vi "Accumet 50 Serial Port Init.vi"(1 "flow control etc.":T1={"input XON/XOFF"=FALSE, "input HW Handshake"=FALSE, "input alt HW HShk"=FALSE, "output XON/XOFF"=FALSE, "output HW Handshake"=FALSE, "output alt HW HShk"=FALSE, "XOFF byte "=19, "XON byte"=17, "parity error byte"=0} {"parity error byte" format="%.0x"; "XON byte" format="%.0x"; "XOFF byte" format="%.0x"}, 2 "parity":u16(ring) items=["no parity", "odd parity", "even parity", "mark parity", "space parity"], 3 "buffer size":u16=10000, 4 "stop bits":u16(ring) items=["1 bit", "1.5 bits", "2 bits"], 5 "data bits":u16=8 min=5 max=8 step=1, 6 "baud rate":u16=9600, 7 "port number":i32=1) -> (0 "error code":i32)   [LabVIEW 2010]
doc: "Initializes the selected serial port to the specified settings."
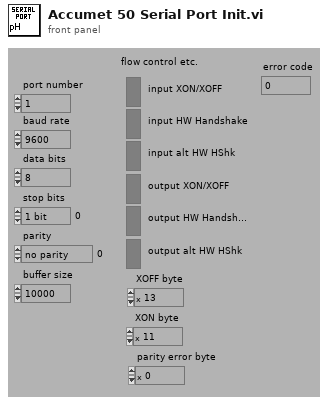
[diagram p1: front panel]
types:
  T1 = cluster{"input XON/XOFF":bool, "input HW Handshake":bool, "input alt HW HShk":bool, "output XON/XOFF":bool, "output HW Handshake":bool, "output alt HW HShk":bool, "XOFF byte ":u8, "XON byte":u8, "parity error byte":u16}
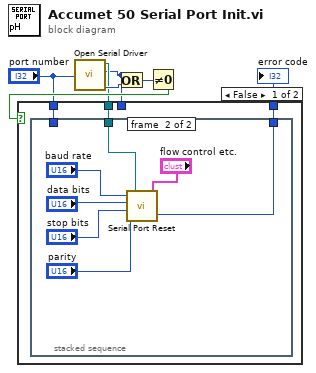
[diagram p0: block diagram]
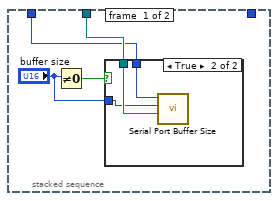
[diagram p2: hidden frame]
diagram:
  n1 = call <vilib>:"Open Serial Driver.vi"("port number"="port number") -> ("input refnum"=w4:refnum<visa-resource-name>, "input error"=w2:i32, "output error"=w6:i32)  [unwired: 1 out]
  n2 = Or(x=w2, y=w6) -> (x .or. y?=w7:i32)
  n3 = Not Equal To 0?(x=w7) -> (x != 0?=w5:bool)
  n4 = case shown="False" w5 {
    tunnel: w4 -> [w10 _]
    tunnel: [w9 w25] -> w3
    tunnel: w2 -> [_ w25]
    tunnel: "port number" -> [w8 _]
    frame False {
      n5 = stacked-sequence {
        tunnel: w10 -> [w12 w24]
        tunnel: [_ w20] -> w9
        tunnel: w8 -> [w11 _]
        frame #0 {
          n6 = Not Equal To 0?(x="buffer size") -> (x != 0?=w14:bool)
          n7 = case shown="True" w14 {
            tunnel: "buffer size" -> [_ w16]
            tunnel: w12 -> [_ w17]
            tunnel: w11 -> [_ w15]
            frame False {
            }
            frame True {
              n8 = call <vilib>:"Serial Port Buffer Size.vi"("in ref"=w17, "buffer size"=w16, "port number (unused)"=w15) -> ()  [unwired: 1 in, 1 out]
            }
          }
        }
        frame #1 {
          n9 = call <vilib>:"Serial Port Reset.vi"("flow control etc."="flow control etc.", "input refnum"=w24, "parity"="parity", "stop bits"="stop bits", "data bits"="data bits", "baud rate"="baud rate") -> ("error"=w20:i32)  [unwired: 1 in]
        }
      }
    }
    frame True {
    }
  }
  "error code" <- w3
